vi "LVClass_WavefrontCorrector Set Actuator Preferences.vi"(0 "WavefrontCorrector in":refnum<class "WavefrontCorrector.lvclass">, 5 "Index of actuator":i32, 7 "Wavefront Corrector state":T1, 11 "error in (no error)":errorcluster) -> (4 "WavefrontCorrector out":refnum<class "WavefrontCorrector.lvclass">, 15 "error out":errorcluster)   [LabVIEW 2020, in "WavefrontCorrector.lvclass"]
uses:
  WavefrontCorrector.lvclass
  Wavefront Corrector states - ONE.ctl
  WavefrontCorrector.lvclass/WavefrontCorrector.ctl
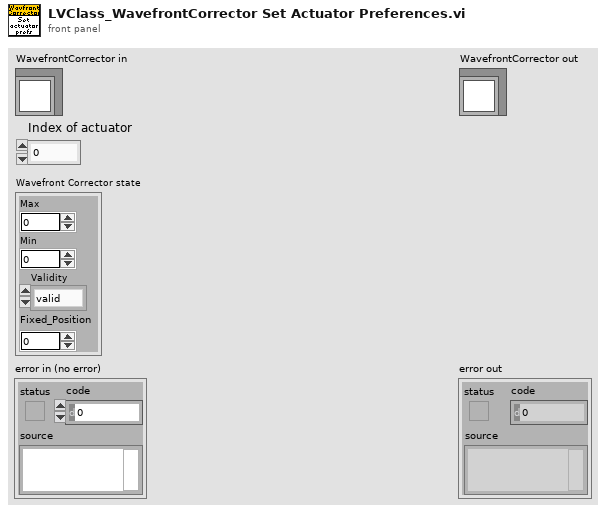
[diagram p1: front panel]
types:
  T1 = typedef "Wavefront Corrector states - ONE.ctl" = cluster{"Max":sgl, "Min":sgl, "Validity":enum16{"valid", "fixed", "invalid"}, "Fixed_Position":sgl}
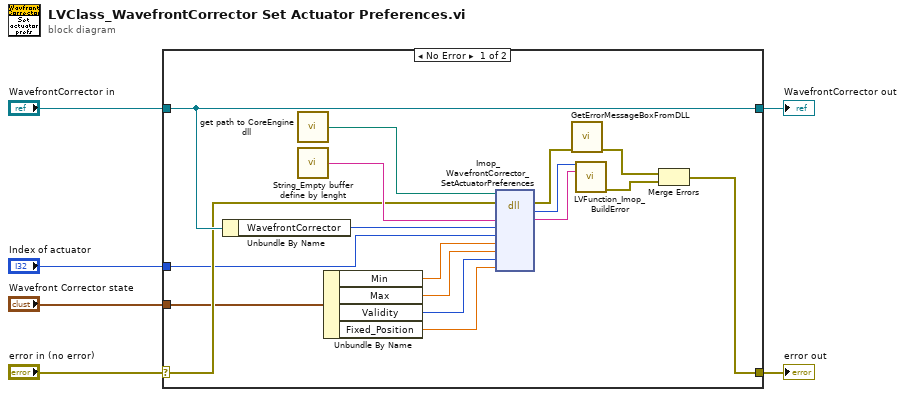
[diagram p0: block diagram]
diagram:
  n1 = case shown="No Error" "error in (no error)" {
    selector: "error in (no error)" -> [w14 w25]
    tunnel: [w13 w25] -> w5
    tunnel: [w15 w24] -> w3
    tunnel: "WavefrontCorrector in" -> [w15 w24]
    tunnel: "Wavefront Corrector state" -> [w12 _]
    tunnel: "Index of actuator" -> [w7 _]
    frame No Error {
      n2 = Unbundle By Name(w15) -> ("WavefrontCorrector"=w21:i32)
      n3 = call "get path to CoreEngine dll.vi"() -> ("path to c_interface_vc100.dll"=w23:path)  [unwired: 12 in, 3 out]
      n4 = call "String_Empty buffer define by lenght.vi"() -> ("Empty buffer"=w22:string)  [unwired: 1 in]
      n5 = Unbundle By Name(w12) -> ("Min"=w11:sgl, "Max"=w10:sgl, "Validity"=w9:enum16{"valid", "fixed", "invalid"}, "Fixed_Position"=w8:sgl)
      n6 = dll-call lib="D:/FLE/0.Code/CoreEngine4_Suite/LV2011_interface/DLLs/c_interface_vc100.dll" fn="Imop_WavefrontCorrector_SetActuatorPreferences"(path in=w23, error in=w14, "Message"=w22, "Wavefront Corrector"=w21, "Index of actuator"=w7, "Min"=w11, "Max"=w10, "Validity"=w9, "Fixed_positions"=w8) -> (error out=w20:errorcluster, "return type"=w18:i32, "Message"=w17:string)  [unwired: 7 in, 1 out]
      n7 = call "GetErrorMessageBoxFromDLL.vi"("error IN"=w20) -> ("error OUT"=w19:errorcluster)  [unwired: 10 in]
      n8 = call "LVFunction_Imop_BuildError.vi"("code"=w18, "String to Prepend to source (\"\")"=w17) -> ("error out"=w16:errorcluster)  [unwired: 13 in]
      n9 = Merge Errors(w19, w16) -> (w13:errorcluster)
    }
    frame Error {
    }
  }
  "error out" <- w5
  "WavefrontCorrector out" <- w3
